vi "MoveSubPanelsToSide.vi"(8 "error in (no error)":errorcluster, 11 "VI Name (Empty = Caller)":string) -> (0 "error out":errorcluster)   [LabVIEW 2012]
uses:
  <vilib>/Utility/miscctls.llb/LVBoundsTypeDef.ctl
  <vilib>/Utility/miscctls.llb/LVPositionTypeDef.ctl
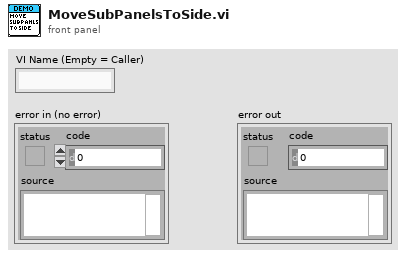
[diagram p1: front panel]
types:
  T1 = typedef "LVPositionTypeDef.ctl" = cluster{"Left":i32, "Top":i32}
  T2 = typedef "LVBoundsTypeDef.ctl" = cluster{"Width":u32, "Height":u32}
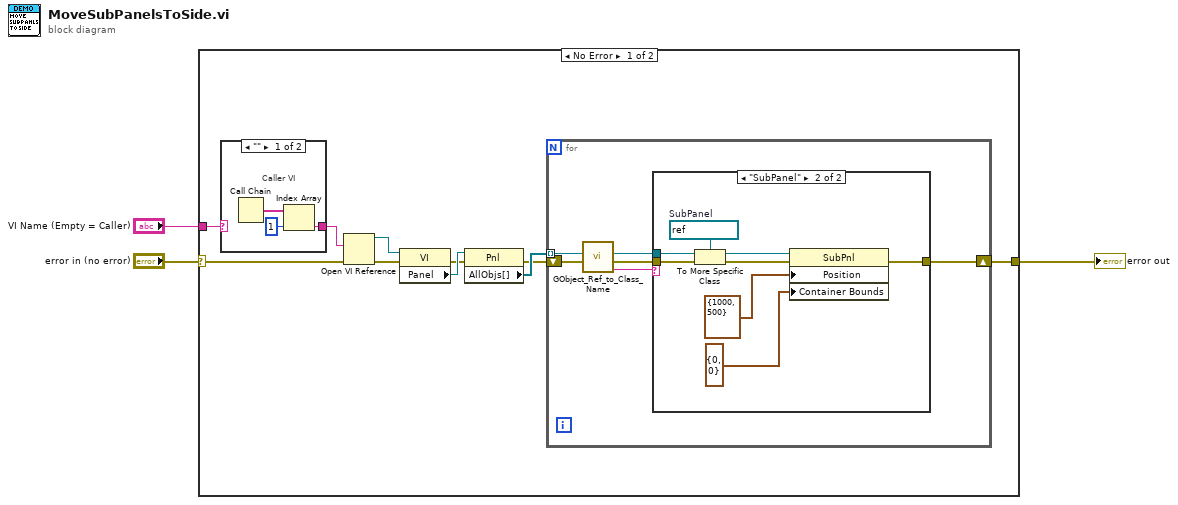
[diagram p0: block diagram]
diagram:
  n1 = case shown="No Error" "error in (no error)" {
    selector: "error in (no error)" -> [w7 w33]
    tunnel: [w9 w33] -> w1
    tunnel: "VI Name (Empty = Caller)" -> [w8 _]
    frame No Error {
      n2 = case shown="\"\"" w8 {
        selector: w8 -> [_ w17]
        tunnel: [w14 w17] -> w5
        frame "" {
          # "Caller VI"
          n3 = Call Chain() -> (call chain=w16:string[])
          n4 = Index Array(array=w16, index=1) -> (element=w14:string)
        }
        frame Default {
        }
      }
      n5 = Open VI Reference(vi path=w5, error in (no error)=w7) -> (vi reference=w4:refnum<vi>, error out=w6:errorcluster)  [unwired: 4 in]
      n6 = property class="VI"(reference=w4, error in=w6) -> (error out=w11:errorcluster, "Panel"=w13:refnum<vi>)  [unwired: 1 out]
      n7 = property class="Pnl"(reference=w13, error in=w11) -> (error out=w10:errorcluster, "AllObjs[]"=w12:refnum<vi>[])  [unwired: 1 out]
      n8 = for {
        tunnel: w12 -> [w22] mode=indexing
        shift-right: [w23] -> w9
        shift-left: w10 -> [w20]
        n9 = call "GObject_Ref_to_Class_Name.vi"("error in"=w20, "GObject Ref In"=w22) -> ("Class Name Out"=w18:string, "error out"=w19:errorcluster, "GObject Ref Out"=w21:refnum<vi>)  [unwired: 7 in]
        n10 = case shown="\"SubPanel\"" w18 {
          tunnel: w19 -> [w24 w31]
          tunnel: w21 -> [_ w32]
          tunnel: [w24 w26] -> w23
          frame Default {
          }
          frame "SubPanel" {
            w30 = refnum<vi> refnum  # SubPanel
            n11 = To More Specific Class(target class=w30, reference=w32, error in=w31) -> (specific class reference=w25:refnum<vi>, error out=w29:errorcluster)
            n12 = property class="SubPnl"(reference=w25, error in=w29, "Position"=T1 {"Left"=1000, "Top"=500}, "Container Bounds"=T2 {"Width"=0, "Height"=0}) -> (error out=w26:errorcluster)  [unwired: 1 out]
          }
        }
      }
    }
    frame Error {
    }
  }
  "error out" <- w1
